vi "demo-ui.vi"() -> ()   [LabVIEW 2018]
uses:
  <vilib>/Utility/miscctls.llb/LVRowAndColumnTypeDef.ctl
panel:
  in  "Integer":i32=12 caption="Numeric"
  in  "Numeric Control":dbl=14.23 format="%#_f"
  in  "Time Stamp":timestamp format="%<%.3X>T\n%<%x>T"
  in  "record?":bool=TRUE
  in  "Tab Control":enum32{"Page 1", "Page 2", "Page 3", "Page 4"}(tab)=enum."Page 2"
  out "Waveform Chart":cluster{dbl, dbl}(graph)={5.001586331627292, 3.0796417607862776}
  in  "DAQmx Physical Channel":tag="cDAQ1Mod1/ai0:1"
  out "result":bool=TRUE
  out "Multicolumn Listbox":i32(listbox)=1
  in  "Ring":u16(ring) items=["Item 1"]
  out "error out":errorcluster
  in  "String - Single Line":string="username"
  in  "Horizontal Slide":dbl(slide)=3.823529411764706 scale=0.0..10.0
  in  "print":bool
  in  "refresh":bool
  in  "write":bool
  in  "settings":bool
  in  "Switch":bool
  in  "Settings":bool
  in  "Close":bool
  in  "header":bool
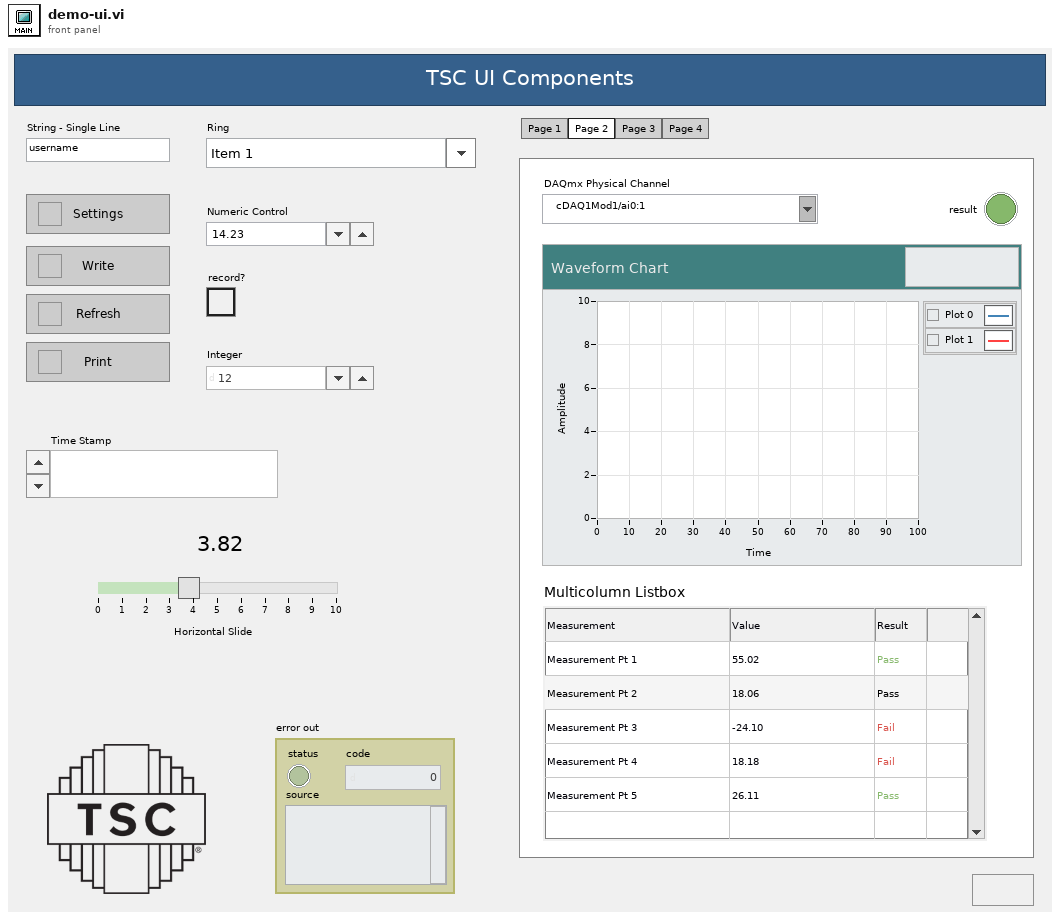
[diagram p1: front panel]
types:
  T1 = typedef "LVRowAndColumnTypeDef.ctl" = cluster{"Row":i32, "Column":i32}
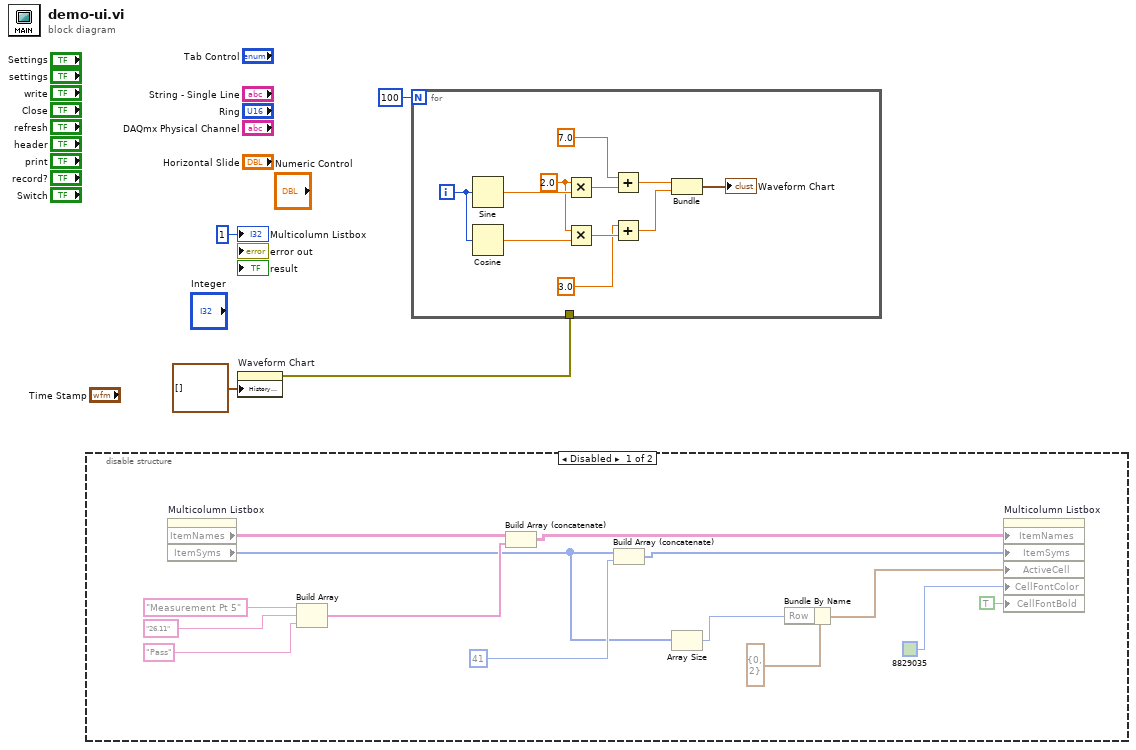
[diagram p0: block diagram]
diagram:
  n1 = disable-structure shown="Disabled" {
    frame Disabled {
      n2 = property on="Multicolumn Listbox" class="MCListbox (strict)"() -> ("ItemNames"=w18:string[][], "ItemSyms"=w10:i32[])  [unwired: 2 in, 2 out]
      n3 = Build Array("Measurement Pt 5" ("String"), "26.11" ("String"), "Pass" ("String")) -> (w13:string[])
      n4 = Build Array (concatenate)(w18, w13) -> (w17:string[][])
      n5 = Build Array (concatenate)(w10, 41) -> (w12:i32[])
      n6 = Array Size(array=w10) -> (size(s)=w8:i32)
      n7 = Bundle By Name(cluster=T1 {"Row"=0, "Column"=2} ("Active Cell:Active Cell"), "Row"=w8) -> (w7:T1)
      n8 = property on="Multicolumn Listbox" class="MCListbox (strict)"("ItemNames"=w17, "ItemSyms"=w12, "ActiveCell"=w7, "CellFontColor"=u32 8829035, "CellFontBold"=TRUE ("Active Cell:Cell Font:Bold")) -> ()  [unwired: 2 in, 2 out]
    }
    frame Enabled {
    }
  }
  n9 = property on="Waveform Chart" class="WFChart (strict)"("History Data"=cluster{dbl, dbl}[] []) -> (error out=w3:errorcluster)  [unwired: 2 in, 1 out]
  n10 = for {
    N: 100 -> [_]
    tunnel: w3 -> [_]
    i -> [w26]
    w22 = 2.0 ("x")
    n11 = Sine(x=w26) -> (sin(x)=w29:dbl)
    n12 = Cosine(x=w26) -> (cos(x)=w21:dbl)
    n13 = Multiply(x=w22, y=w29) -> (x*y=w28:dbl)
    n14 = Multiply(x=w22, y=w21) -> (x*y=w24:dbl)
    n15 = Add(x=7.0, y=w28) -> (x+y=w27:dbl)
    n16 = Add(x=3.0, y=w24) -> (x+y=w23:dbl)
    n17 = Bundle(w27, w23) -> (→"Waveform Chart":cluster{dbl, dbl})  [unwired: 1 in]
  }
  "Multicolumn Listbox" <- 1 ("Multicolumn Listbox")
